vi "rqcBob Wait Until Done.vi"(0 "rqcBob in":refnum<class "rqcBob.lvclass">, 5 "Timeout (ms)":u32=1000, 11 "error in (no error)":errorcluster) -> (4 "rqcBob out":refnum<class "rqcBob.lvclass">, 15 "error out":errorcluster)   [LabVIEW 2019, in "rqcBob.lvclass"]
uses:
  rqcBob.lvclass
  <vilib>/Utility/error.llb/Error Cluster From Error Code.vi
  <vilib>/ErrorRing/Error Ring.xnode
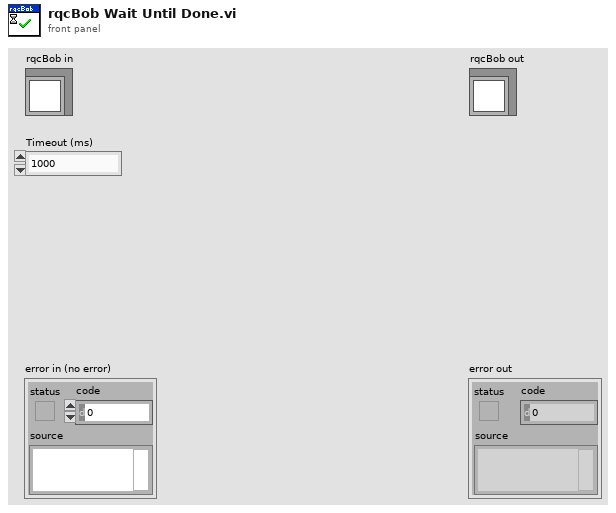
[diagram p1: front panel]
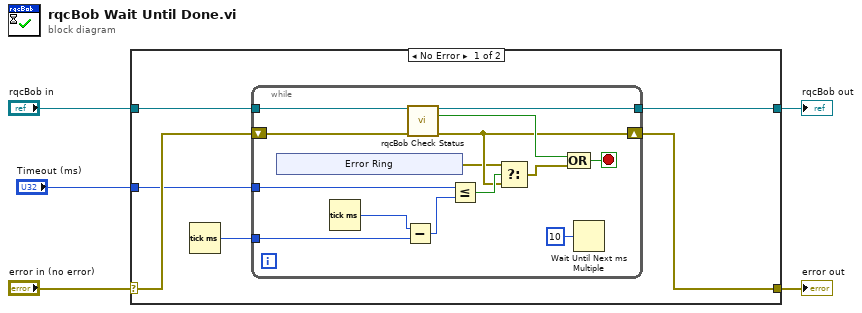
[diagram p0: block diagram]
diagram:
  n1 = case shown="No Error" "error in (no error)" {
    selector: "error in (no error)" -> [w9 w32]
    tunnel: [w8 w32] -> w4
    tunnel: [w10 w31] -> w2
    tunnel: "rqcBob in" -> [w11 w31]
    tunnel: "Timeout (ms)" -> [w6 _]
    frame No Error {
      n2 = Tick Count (ms)() -> (millisecond timer value=w7:u32)
      n3 = while {
        tunnel: w11 -> [w25]
        tunnel: [w24] -> w10
        shift-right: [w15] -> w8
        shift-left: w9 -> [w23]
        tunnel: w7 -> [w21]
        tunnel: w6 -> [w18]
        stop <- w12 stop-if-true
        n4 = xnode "Error Ring"() -> ("error out"=w14:errorcluster)
        n5 = Tick Count (ms)() -> (millisecond timer value=w20:u32)
        n6 = Subtract(x=w20, y=w21) -> (x-y=w19:u32)
        n7 = call-dynamic "rqcBob Check Status.vi"("rqcBob in"=w25, "error in (no error)"=w23) -> ("rqcBob out"=w24:refnum<class "rqcBob.lvclass">, "done?"=w16:bool, "error out"=w15:errorcluster)  [unwired: 11 in]
        n8 = Less Or Equal?(x=w18, y=w19) -> (x <= y?=w17:bool)
        n9 = Select(t=w14, s=w17, f=w15) -> (s? t:f=w13:errorcluster)
        n10 = Compound Arithmetic op=OR(w16, w13) -> (w12:bool)
        n11 = Wait Until Next ms Multiple(millisecond multiple=u32 10) -> ()  [unwired: 1 out]
      }
    }
    frame Error {
    }
  }
  "error out" <- w4
  "rqcBob out" <- w2
